vi "selectAutonMode.vi"(1 "Joystick":bool) -> ()   [LabVIEW 2011]
uses:
  <vilib>/Rock Robotics/WPI/DriverStation/DriverStationLCD/WPI_DriverStationLCDLCDLine.ctl
  Robot Global Data.vi
panel:
  in  "File Number":dbl
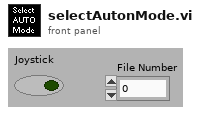
[diagram p1: front panel]
types:
  T1 = typedef "WPI_DriverStationLCDLCDLine.ctl" = enum16{"Main - Line 1", "User - Line 2", "User - Line 3", "User - Line 4", "User - Line 5", "User - Line 6"}
  T2 = enum16{"False", "FalseToTrue", "True", "TrueToFalse"}
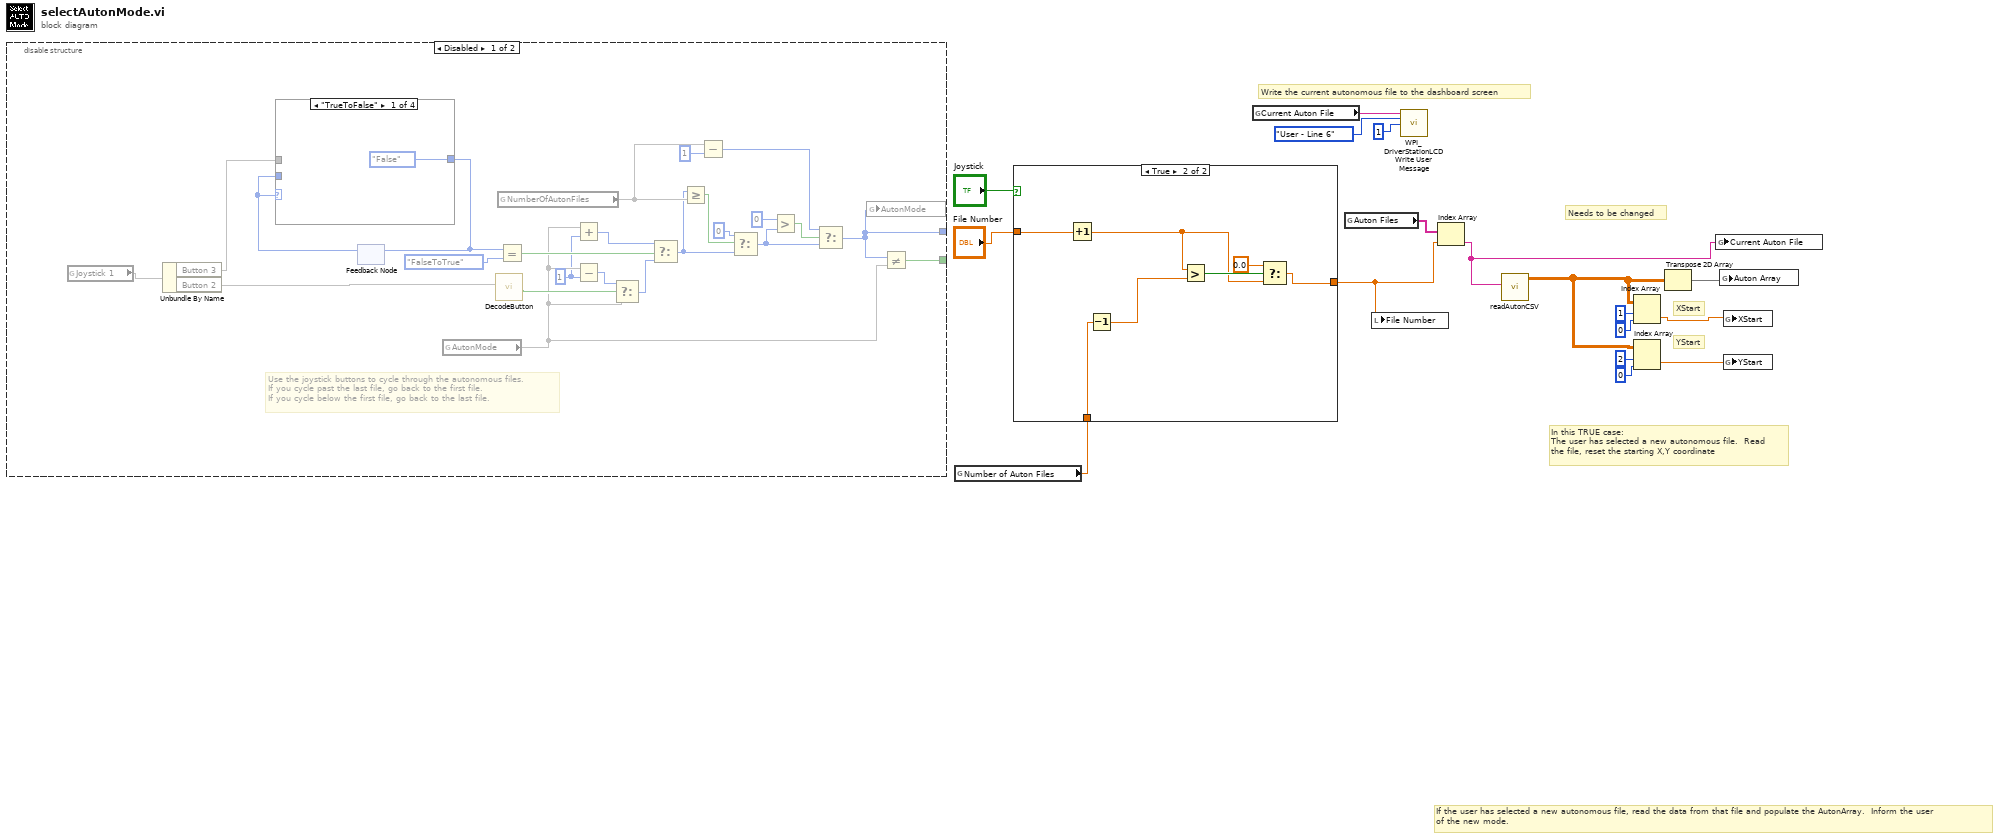
[diagram p0: block diagram]
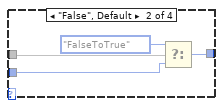
[diagram p3: hidden frame]
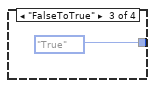
[diagram p4: hidden frame]
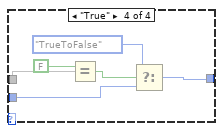
[diagram p5: hidden frame]
diagram:
  # "Needs to be changed"
  # "In this TRUE case:\nThe user has selected a new autonomous file.  Read\nthe file, reset the starting X,Y coordinate"
  # "YStart"
  # "XStart"
  # "Write the current autonomous file to the dashboard screen"
  # "If the user has selected a new autonomous file, read the data from that file and populate the AutonArray.  Inform the user\nof the new mode."
  n1 = disable-structure shown="Disabled" {
    disable-tunnel: [w41 _] -> _
    disable-tunnel: [w31 _] -> _
    frame Disabled {
      w22 = i16 1 ("y")
      # "Use the joystick buttons to cycle through the autonomous files.\nIf you cycle past the last file, go back to the first file.\nIf you cycle below the first file, go back to the last file."
      n2 = global read "Robot Global Data.vi" "Joystick 1"() -> (w18)
      n3 = Unbundle By Name(w18) -> ("Button 3"=w29, "Button 2"=w19)
      n4 = feedback #1() -> (w26:T2)  [unwired: 1 out]
      n5 = case shown="\"TrueToFalse\"" w26 {
        tunnel: w29 -> [_ w46 _ w52]
        tunnel: [T2."False" ("f") w44 T2."True" ("y") w53] -> w27
        tunnel: w26 -> [_ w43 _ w49]
        frame "TrueToFalse" {
        }
        frame "False", Default {
          n6 = Select(t=T2."FalseToTrue", s=w46, f=w43) -> (s? t:f=w44:T2)
        }
        frame "FalseToTrue" {
        }
        frame "True" {
          n7 = Equal?(x=FALSE, y=w52) -> (x = y?=w50:bool)
          n8 = Select(t=T2."TrueToFalse", s=w50, f=w49) -> (s? t:f=w53:T2)
        }
      }
      n9 = feedback-in #1(w27) -> ()
      n10 = global read "Robot Global Data.vi" "AutonMode"() -> (w24)
      n11 = call "DecodeButton.vi"("Button"=w19) -> ("False to True"=w25:bool)  [unwired: 10 out]
      n12 = global read "Robot Global Data.vi" "NumberOfAutonFiles"() -> (w38)
      n13 = Equal?(x=w27, y=T2."FalseToTrue") -> (x = y?=w30:bool)
      n14 = Add(x=w24, y=w22) -> (x+y=w23:i16)
      n15 = Subtract(x=w24, y=w22) -> (x-y=w20:i16)
      n16 = Select(t=w20, s=w25, f=w24) -> (s? t:f=w21:i16)
      n17 = Select(t=w23, s=w30, f=w21) -> (s? t:f=w32:i16)
      n18 = Greater Or Equal?(x=w32, y=w38) -> (x >= y?=w33:bool)
      n19 = Subtract(x=w38, y=i16 1) -> (x-y=w40:i16)
      n20 = Select(t=i16 0, s=w33, f=w32) -> (s? t:f=w35:i16)
      n21 = Greater?(x=i16 0, y=w35) -> (0:w37:bool)
      n22 = Select(t=w40, s=w37, f=w35) -> (s? t:f=w41:i16)
      n23 = global write "Robot Global Data.vi" "AutonMode"(w41) -> ()
      n24 = Not Equal?(x=w41, y=w24) -> (x != y?=w31:bool)
    }
    frame Enabled {
    }
  }
  n25 = global read "Robot Global Data.vi" "Number of Auton Files"() -> (w9:dbl)
  n26 = case shown="True" "Joystick" {
    tunnel: "File Number" -> [w54 w61]
    tunnel: [w54 w57] -> w8
    tunnel: w9 -> [_ w56]
    frame False {
    }
    frame True {
      n27 = Increment(x=w61) -> (x+1=w59:dbl)
      n28 = Decrement(x=w56) -> (x-1=w55:dbl)
      n29 = Greater?(x=w59, y=w55) -> (0:w60:bool)
      n30 = Select(t=0.0, s=w60, f=w59) -> (s? t:f=w57:dbl)
    }
  }
  n31 = global read "Robot Global Data.vi" "Current Auton File"() -> (w7:string)
  n32 = global read "Robot Global Data.vi" "Auton Files"() -> (w6:string[])
  n33 = local write "File Number"(w8) -> ()
  n34 = call <vilib>:"WPI_DriverStationLCDWrite User Message.vi"("line text"=w7, "line"=WPI_DriverStationLCDLCDLine."User - Line 6", "starting column"=i8 1) -> ()  [unwired: 2 in, 11 out]
  n35 = Index Array(array=w6, index=w8) -> (element=w3:string)
  n36 = call "readAutonCSV.vi"("AutonFile"=w3) -> ("AutonArray"=w2:dbl[][])  [unwired: 7 out]
  n37 = Index Array(array=w2, index (row)=1 ("disabled index (row)"), index (col)=0) -> (element=w5:dbl)
  n38 = Index Array(array=w2, index (row)=2 ("disabled index (row)"), index (col)=0) -> (element=w4:dbl)
  n39 = Transpose 2D Array(2D array=w2) -> (transposed array=w1:dbl[][])
  n40 = global write "Robot Global Data.vi" "Current Auton File"(w3) -> ()
  n41 = global write "Robot Global Data.vi" "Auton Array"(w1) -> ()
  n42 = global write "Robot Global Data.vi" "XStart"(w5) -> ()
  n43 = global write "Robot Global Data.vi" "YStart"(w4) -> ()
